vi "Test Honeywell HMC6352.vi"() -> (3 "Heading (degrees)":dbl)   [LabVIEW 2011]
uses:
  <vilib>/robotics/Controls/Compass Indicator/Compass Indicator.xctl
  <vilib>/LabVIEW Interface for Arduino/LabVIEW Interface for Arduino.lvlib
panel:
  out "Compass Indicator":dbl(xcontrol)
  in  "stop":bool
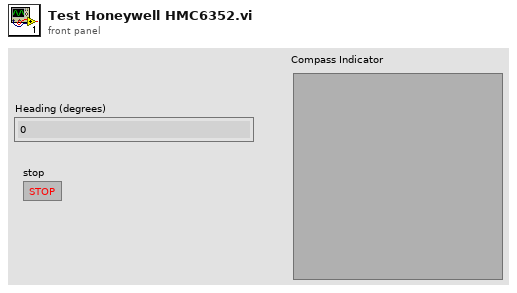
[diagram p1: front panel]
types:
  T1 = typedef "LabVIEW Interface for Arduino.lvlib/Arduino Resource.ctl" = cluster{"VISA resource":refnum<visa-resource-name>, "Board Type":T2, "Connection Type":enum8{"USB / Serial"}, "Bytes Per Packet (15)":u8}
  T2 = typedef "LabVIEW Interface for Arduino.lvlib/Board Type.ctl" = enum16{"Uno", "Dimuelanove w/Atmega 328", "Mega 2560"}
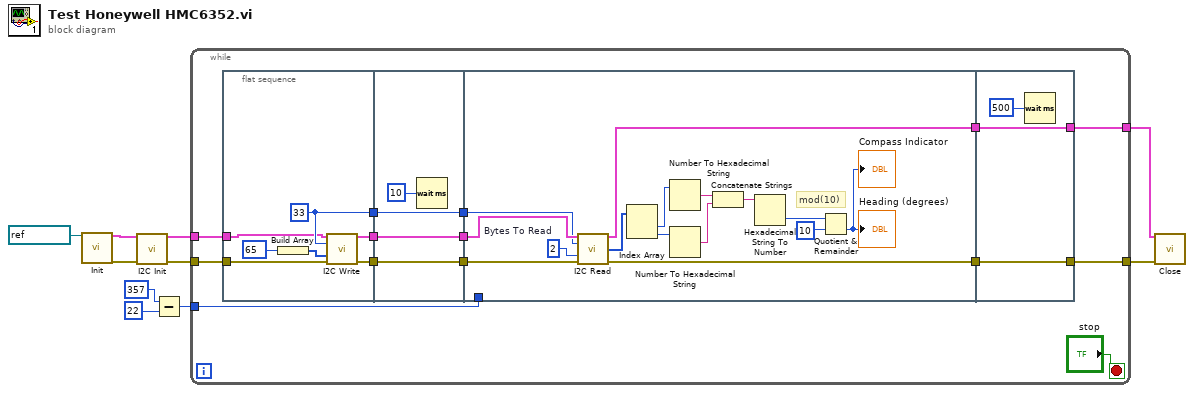
[diagram p0: block diagram]
diagram:
  n1 = call <vilib>:"Init.vi"("VISA resource"=refnum<visa-resource-name> "COM6") -> ("Arduino Resource"=w8:T1, "error out"=w7:errorcluster)  [unwired: 17 in]
  n2 = call <vilib>:"I2C Init.vi"("Arduino Resource"=w8, "error in"=w7) -> ("Arduino Resource"=w6:T1, "error out"=w5:errorcluster)  [unwired: 12 in]
  n3 = Subtract(x=357, y=22) -> (x-y=w1:i32)
  n4 = while {
    tunnel: [w18] -> w10
    tunnel: [w17] -> w9
    tunnel: w6 -> [w15]
    tunnel: w5 -> [w14]
    tunnel: w1 -> [w11]
    stop <- "stop" stop-if-true
    n5 = flat-sequence {
      tunnel: [w31] -> w24
      tunnel: [w30] -> w23
      tunnel: [w27] -> w22
      tunnel: w15 -> [w26]
      tunnel: w14 -> [w25]
      tunnel: [w34] -> w21
      tunnel: w24 -> [w34]
      tunnel: [w33] -> w20
      tunnel: w23 -> [w33]
      tunnel: [w32] -> w19
      tunnel: w22 -> [w32]
      tunnel: w21 -> [w43]
      tunnel: w20 -> [w42]
      tunnel: w19 -> [w38]
      tunnel: [w40] -> w13
      tunnel: [w39] -> w12
      tunnel: w11 -> [_]
      tunnel: [w52] -> w17
      tunnel: [w53] -> w18
      tunnel: w13 -> [w53]
      tunnel: w12 -> [w52]
      frame #0 {
        w27 = u8 33 ("Address (0)")
        n6 = Build Array(u8 65 ("Address (0)")) -> (w29:u8[])
        n7 = call <vilib>:"I2C Write.vi"("Arduino Resource"=w26, "Address (0)"=w27, "I2C Data Bytes"=w29, "error in"=w25) -> ("Arduino Resource"=w31:T1, "error out"=w30:errorcluster)  [unwired: 10 in]
      }
      frame #1 {
        n8 = Wait (ms)(milliseconds to wait=u32 10) -> ()  [unwired: 1 out]
      }
      frame #2 {
        w41 = u8 2  # Bytes To Read
        # "mod(10)"
        n9 = call <vilib>:"I2C Read.vi"("Arduino Resource"=w43, "Address (0)"=w38, "Bytes To Read"=w41, "error in"=w42) -> ("Arduino Resource"=w40:T1, "I2C Data"=w37:u8[], "error out"=w39:errorcluster)  [unwired: 9 in]
        n10 = Index Array(array=w37) -> (element #1=w50:u8, element #2=w49:u8)  [unwired: 2 in]
        n11 = Number To Hexadecimal String(2:w50) -> (0:w45:string)  [unwired: 1 out]
        n12 = Number To Hexadecimal String(2:w49) -> (0:w46:string)  [unwired: 1 out]
        n13 = Concatenate Strings(w45, w46) -> (w44:string)
        n14 = Hexadecimal String To Number(string=w44) -> (number=w47:u32)  [unwired: 3 out]
        n15 = Quotient & Remainder(x=w47, y=10) -> (floor(x/y)=→"Heading (degrees)" →"Compass Indicator":u32)  [unwired: 1 out]
      }
      frame #3 {
        n16 = Wait (ms)(milliseconds to wait=u32 500) -> ()  [unwired: 1 out]
      }
    }
  }
  n17 = call <vilib>:"Close.vi"("Arduino Resource"=w10, "error in"=w9) -> ()  [unwired: 13 in, 1 out]
